vi "Inject Force Tag.vi"(1 "Tag":string="<None>", 2 "Transactions In":T1[](array[typedef])) -> (0 "Transactions Out":T1[](array[typedef]))   [LabVIEW 2009]
uses:
  Dataset Transaction Id.ctl
  Dataset Source.ctl
  Dataset Type.ctl
  Apps/Yes No Button.ctl
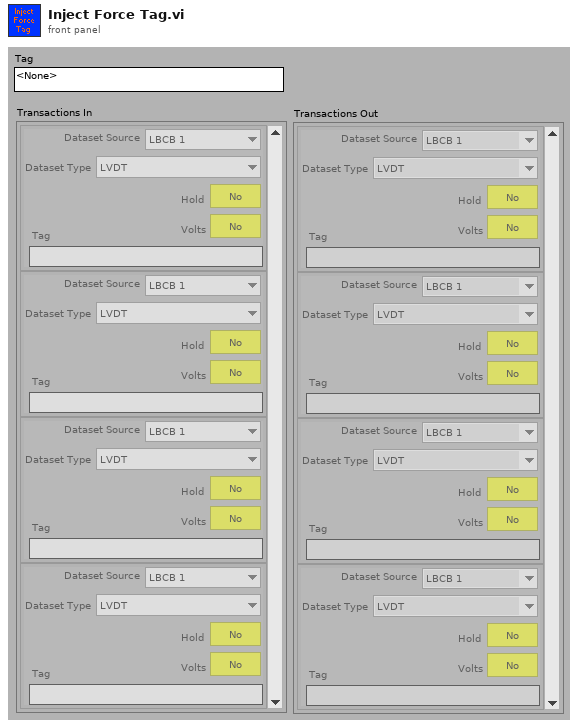
[diagram p1: front panel]
types:
  T1 = typedef "Dataset Transaction Id.ctl" = cluster{"Dataset Source":T2, "Dataset Type":T3, "Hold":T4, "Volts":T4, "Tag":string}
  T2 = typedef "Dataset Source.ctl" = enum16{"LBCB 1", "LBCB 2", "Combined", "External Sensors"}
  T3 = typedef "Dataset Type.ctl" = enum16{"LVDT", "Load Cell", "Actuator Command", "Servo Error", "Displacement Command", "Displacement", "Force"}
  T4 = typedef "Yes No Button.ctl" = bool
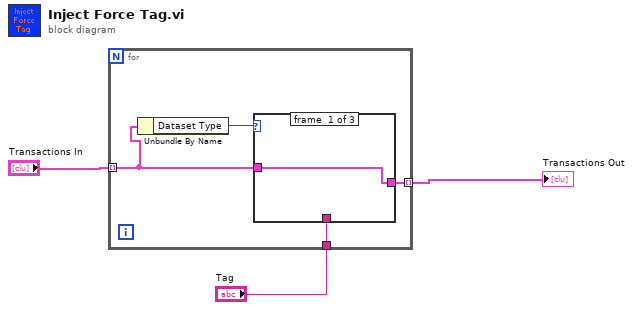
[diagram p0: block diagram]
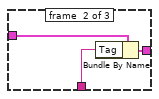
[diagram p2: hidden frame]
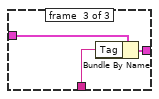
[diagram p3: hidden frame]
diagram:
  n1 = for {
    tunnel: "Transactions In" -> [w5] mode=indexing
    tunnel: [w7] -> w2 mode=indexing
    tunnel: "Tag" -> [w6]
    n2 = Unbundle By Name(w5) -> ("Dataset Type"=w4:T3)
    n3 = case shown="\"Force\"" w4 {
      tunnel: w5 -> [w8 w11 w14]
      tunnel: [w8 w10 w13] -> w7
      tunnel: w6 -> [_ w9 w12]
      frame #0 {
      }
      frame #1 {
        n4 = Bundle By Name(cluster=w11, "Tag"=w9) -> (w10:T1)
      }
      frame #2 {
        n5 = Bundle By Name(cluster=w14, "Tag"=w12) -> (w13:T1)
      }
    }
  }
  "Transactions Out" <- w2
